vi "Throw Error - Impossible Initial State - Reason 2.vi"(8 "error in":errorcluster) -> (0 "error out":errorcluster)   [LabVIEW 2022 SP3]
doc: "Throws a user-generated error that indicates that an impossible initial state was detected."
panel:
  # "Development\ncontrols/indicators useful for development and testing, but which are not outputs of the VI"
  # "Input\nInputs to the VI"
  # "Output\nOutputs of the VI"
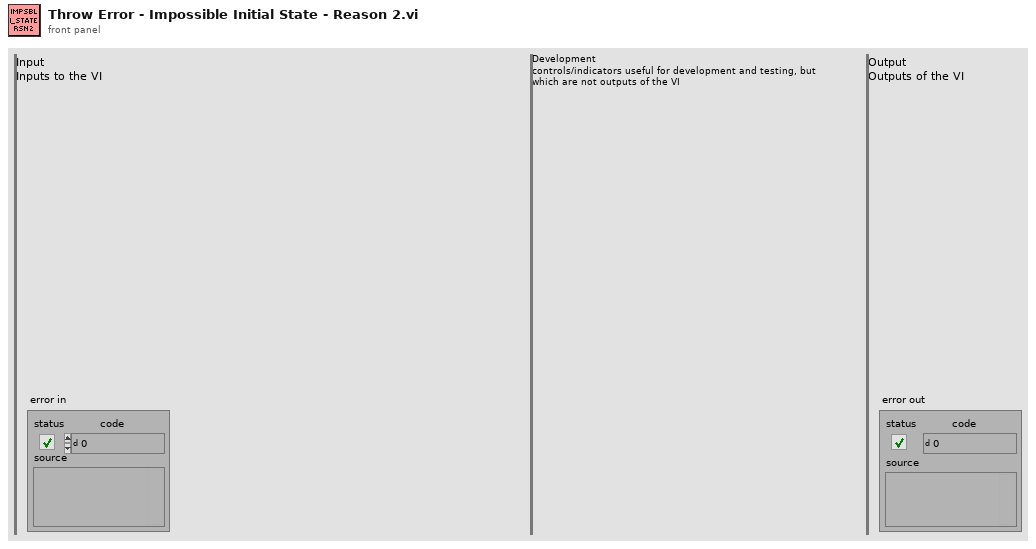
[diagram p1: front panel]
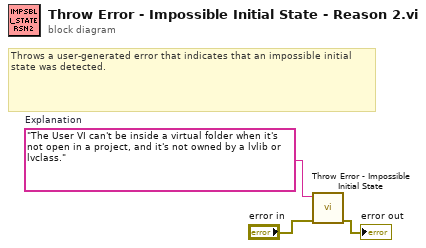
[diagram p0: block diagram]
diagram:
  w3 = "The User VI can't be inside a virtual folder when it's not open in a project, and it's not owned by a lvlib or lvclass."  # Explanation
  # "Throws a user-generated error that indicates that an impossible initial state was detected."
  n1 = call "Throw Error - Impossible Initial State.vi"("error in"="error in", "Explanation"=w3) -> ("error out"=→"error out":errorcluster)  [unwired: 9 in]
